vi "Close.vi"(8 "error in (no error)":errorcluster, 11 "SV B-M (Target) in":refnum<class "SV B-M (Target).lvclass">) -> (0 "error out":errorcluster, 3 "SV B-M (Target) out":refnum<class "SV B-M (Target).lvclass">)   [LabVIEW 2015, in "SV B-M (Target).lvclass"]
uses:
  SV B-M (Target).lvclass
  SV B-M (Target).lvclass/SV B-M (Target).ctl
  Command & Ack - Send Ack.vi
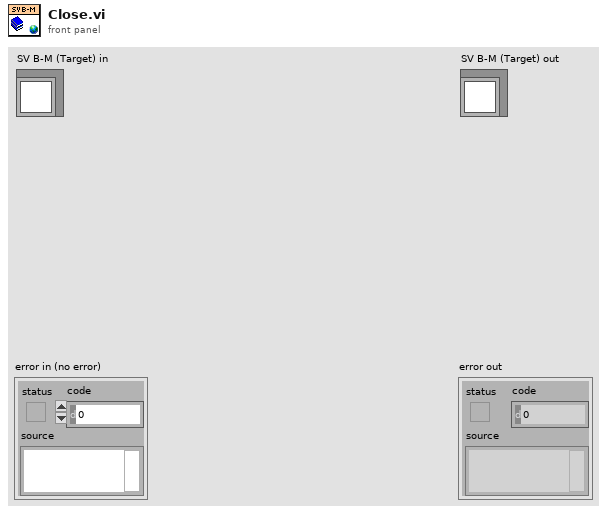
[diagram p1: front panel]
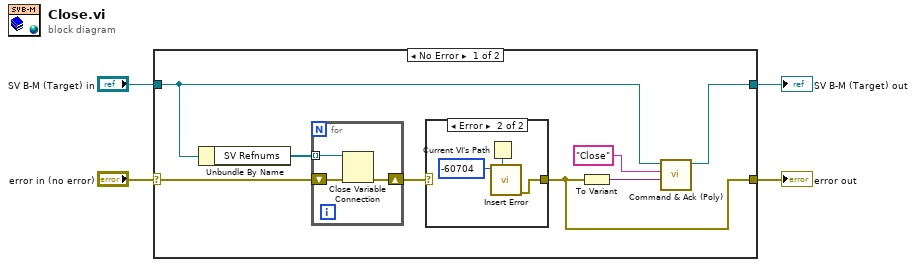
[diagram p0: block diagram]
diagram:
  n1 = case shown="No Error" "error in (no error)" {
    selector: "error in (no error)" -> [w7 w21]
    tunnel: [w5 w21] -> w3
    tunnel: [w10 w20] -> w1
    tunnel: "SV B-M (Target) in" -> [w9 w20]
    frame No Error {
      n2 = Unbundle By Name(w9) -> ("SV Refnums"=w8:refnum<k21>[])
      n3 = for {
        tunnel: w8 -> [w19] mode=indexing
        shift-right: [w17] -> w6
        shift-left: w7 -> [w18]
        n4 = Close Variable Connection(8:w18, 11:w19) -> (0:w17:errorcluster)
      }
      n5 = case shown="Error" w6 {
        selector: w6 -> [w13 _]
        tunnel: [w13 w16] -> w5
        frame No Error {
        }
        frame Error {
          n6 = Current VI's Path() -> (path=w14:path)
          n7 = call "Insert Error.vi"("VI Path"=w14, "Error Code"=-60704) -> ("error out"=w16:errorcluster)  [unwired: 9 in]
        }
      }
      n8 = To Variant(anything=w5) -> (Variant=w12:variant)
      n9 = call-poly "Command & Ack (Poly).vi"("Message Data"=w12, "Message"="Close", "SV B-M (Target) In"=w9) -> ("SV B-M (Target) Out"=w10:refnum<class "SV B-M (Target).lvclass">)  [unwired: 6 in, 2 out]
    }
    frame Error {
    }
  }
  "error out" <- w3
  "SV B-M (Target) out" <- w1
